vi "Returning A Value 2D Array Of Integers.vi"(8 "error in (no error)":errorcluster, 10 "cols":i32, 11 "rows":i32) -> (0 "error out":errorcluster, 3 "function return":i32)   [LabVIEW 2009, in "LabVIEWWrapper_PassingDataSampleDLL.lvlib"]
doc: "int** ReturningAValue_2DArrayOfIntegers (int rows, int cols);"
uses:
  LabVIEWWrapper_PassingDataSampleDLL.lvlib
  PassingDataSampleDLL.dll
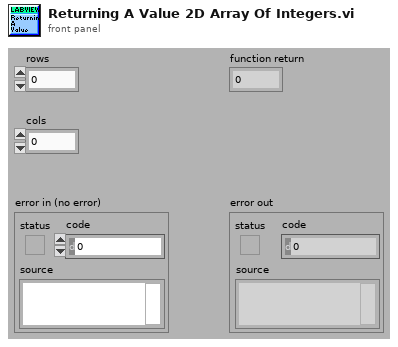
[diagram p1: front panel]
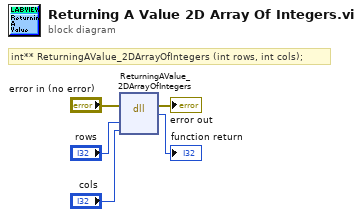
[diagram p0: block diagram]
diagram:
  # "int** ReturningAValue_2DArrayOfIntegers (int rows, int cols);"
  n1 = dll-call lib="C:/My Dropbox/Systems Engineering Application/SDK/C Integration/LabVIEWWrapper/PassingDataSampleDLL.*" fn="ReturningAValue_2DArrayOfIntegers"(error in="error in (no error)", "rows"="rows", "cols"="cols") -> (error out=→"error out":errorcluster, →"function return":i32)  [unwired: 4 in, 1 out]
